vi "_TotalMDptrCount.vi"(8 "error in (no error)":errorcluster, 11 "MDPtrMgr in":refnum<class "MDPtrMgr.lvclass">) -> (0 "error out":errorcluster, 1 "# free elements in queue":i32, 2 "# elements in queue":i32, 3 "MDPtrMgr out":refnum<class "MDPtrMgr.lvclass">, 4 "#queues":i32)   [LabVIEW 2017, in "MDPtr.lvlib" / "MDPtrMgr.lvclass"]
uses:
  MDPtrMgr.lvclass
  MDPtrMgr.lvclass/MDPtrMgr.ctl
  Def-MDPtrQueue.ctl
  MDPtr TypeDef/MDPtr.ctl
  MDPtr.lvlib
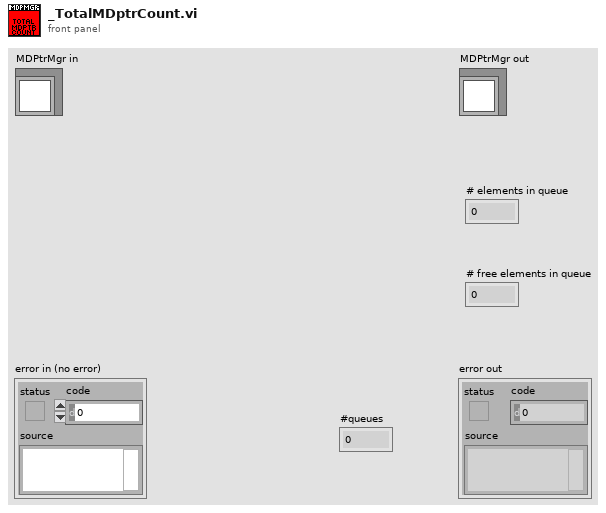
[diagram p1: front panel]
types:
  T1 = typedef "MDPtr.lvlib/Def-MDPtrQueue.ctl" = refnum<queue>
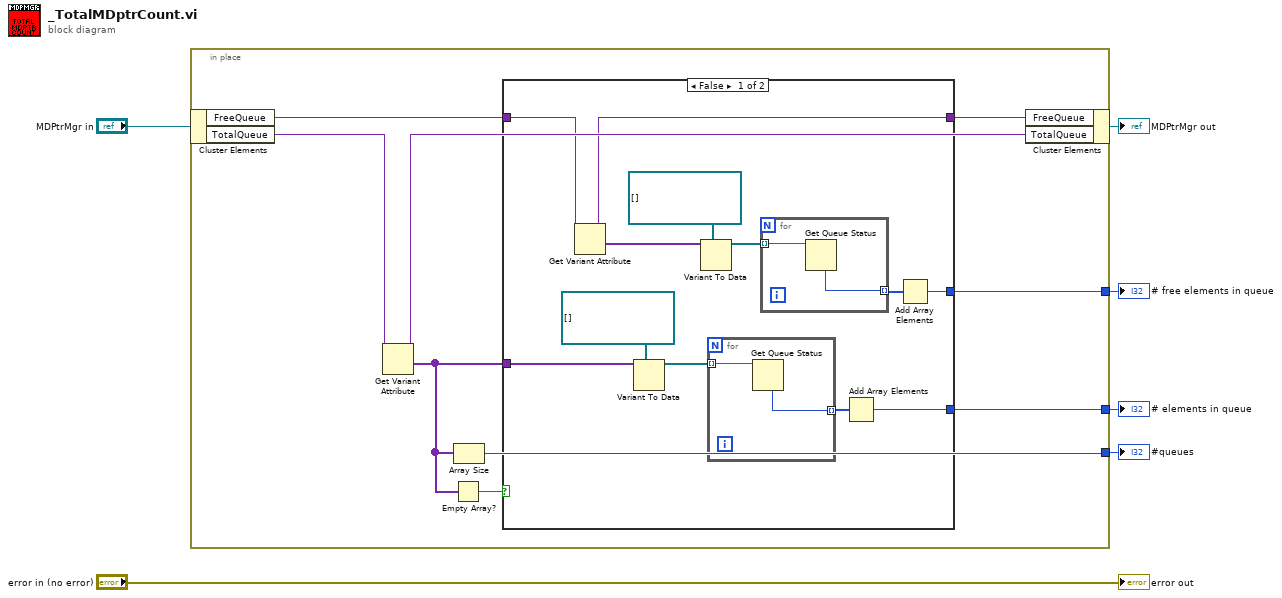
[diagram p0: block diagram]
diagram:
  n1 = in-place "In Place Element Structure" {
    in-place-border: [w13] -> w3
    in-place-border: [w12] -> w2
    in-place-border: [w7] -> w1
    n2 = in-place-cluster #1("MDPtrMgr in") -> ("FreeQueue"=w8:variant, "TotalQueue"=w15:variant)
    n3 = Get Variant Attribute(Variant=w15) -> (duplicate Variant=w14:variant, values=w10:variant[])  [unwired: 3 in, 2 out]
    n4 = Empty Array?(array=w10) -> (empty?=w11:bool)
    n5 = Array Size(array=w10) -> (size(s)=w12:i32)
    n6 = case shown="False" w11 {
      tunnel: [w24 _] -> w13
      tunnel: w10 -> [w23 _]
      tunnel: [w17 w32] -> w9
      tunnel: w8 -> [w18 w32]
      tunnel: [w16 _] -> w7
      frame False {
        n7 = Get Variant Attribute(Variant=w18) -> (duplicate Variant=w17:variant, values=w21:variant[])  [unwired: 3 in, 2 out]
        n8 = Variant To Data(type=T1[] [] ("Array"), Variant=w23) -> (data=w26:T1[])  [unwired: 1 in, 1 out]
        n9 = Variant To Data(type=T1[] [] ("Array"), Variant=w21) -> (data=w20:T1[])  [unwired: 1 in, 1 out]
        n10 = for {
          tunnel: w26 -> [w31] mode=indexing
          tunnel: [w30] -> w25 mode=indexing
          n11 = Get Queue Status(queue=w31) -> (# elements in queue=w30:i32)  [unwired: 2 in, 7 out]
        }
        n12 = for {
          tunnel: w20 -> [w29] mode=indexing
          tunnel: [w28] -> w19 mode=indexing
          n13 = Get Queue Status(queue=w29) -> (# elements in queue=w28:i32)  [unwired: 2 in, 7 out]
        }
        n14 = Add Array Elements(numeric array=w25) -> (sum=w24:i32)
        n15 = Add Array Elements(numeric array=w19) -> (sum=w16:i32)
      }
      frame True {
      }
    }
    n16 = in-place-cluster #1("FreeQueue"=w9, "TotalQueue"=w14) -> (→"MDPtrMgr out":refnum<class "MDPtrMgr.lvclass">)
  }
  "# elements in queue" <- w3
  "#queues" <- w2
  "# free elements in queue" <- w1
  "error out" <- "error in (no error)"
